vi "CANFD Set Filter.vi"(7 "Len":u8, 9 "pCanFilter":T1, 10 "CANIndex":u8, 11 "DevHandle":i32) -> (1 "pCanFilter out":T1, 3 "function return":i32)   [LabVIEW 2010, in "usb2canfd.lvlib"]
doc: "int WINAPI CANFD_SetFilter(int DevHandle, unsigned char CANIndex, CANFD_FILTER_CONFIG *pCanFilter,unsigned char Len);"
uses:
  usb2canfd.lvlib
  USB2XXX/trunk/USB2XXX/USB2XXX/vs2019/Release/USB2XXX.dll
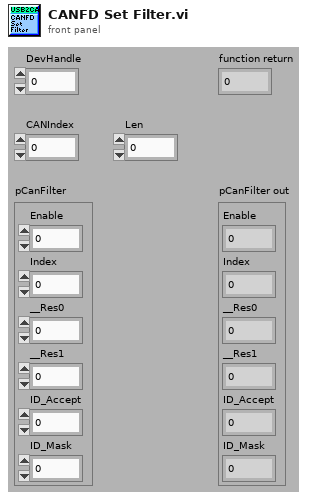
[diagram p1: front panel]
types:
  T1 = cluster{"Enable":u8, "Index":u8, "__Res0":u8, "__Res1":u8, "ID_Accept":u32, "ID_Mask":u32}
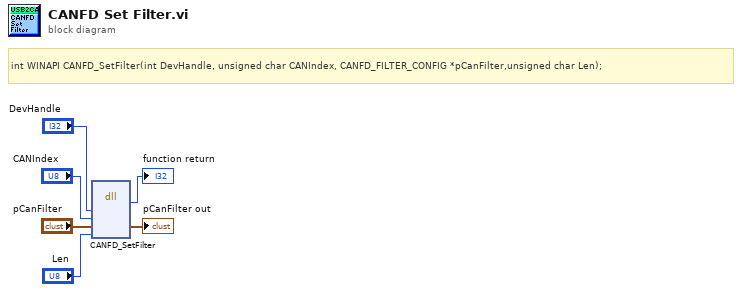
[diagram p0: block diagram]
diagram:
  # "int WINAPI CANFD_SetFilter(int DevHandle, unsigned char CANIndex, CANFD_FILTER_CONFIG *pCanFilter,unsigned char Len);"
  n1 = dll-call lib="E:/Projects/USB2XXX/trunk/USB2XXX/USB2XXX/vs2019/Release/USB2XXX.*" fn="CANFD_SetFilter"("DevHandle"="DevHandle", "CANIndex"="CANIndex", "pCanFilter"="pCanFilter", "Len"="Len") -> (→"function return":i32, "pCanFilter"=→"pCanFilter out":T1)  [unwired: 6 in, 2 out]
